vi "ClawGainScheduler.vi"(10 "On Bert?":bool=TRUE, 11 "Claw States":T2) -> (3 "ClawGainsOut":T1)   [LabVIEW 2014]
uses:
  Typedefs/ClawStates.ctl
panel:
  in  "Claw Gains for Ernie":T1={"Arm_kP"=13.5, "Arm_kI"=0.0, "Arm_kD"=0.0}
  in  "Claw Gains for Bert":T1={"Arm_kP"=10.0, "Arm_kI"=0.0, "Arm_kD"=0.0}
  in  "Claw Gains for Manual":T1
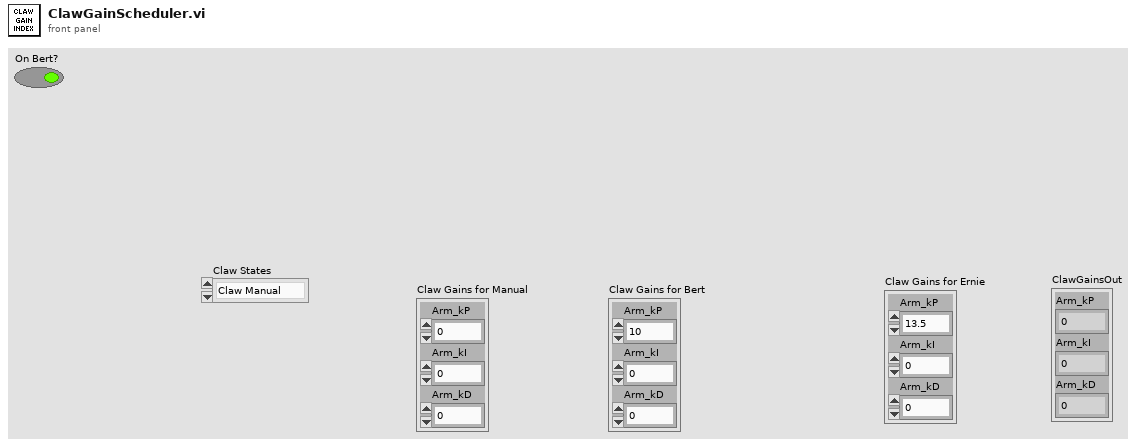
[diagram p1: front panel]
types:
  T1 = cluster{"Arm_kP":dbl, "Arm_kI":dbl, "Arm_kD":dbl}
  T2 = typedef "ClawStates.ctl" = enum16{"Claw Manual ", "Claw Open", "Claw Closed", "Claw Slight Open", "Flip Can"}
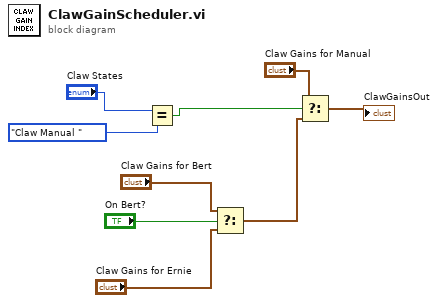
[diagram p0: block diagram]
diagram:
  n1 = Equal?(x="Claw States", y=ClawStates."Claw Manual " ("Claw States")) -> (x = y?=w6:bool)
  n2 = Select(t="Claw Gains for Bert", s="On Bert?", f="Claw Gains for Ernie") -> (s? t:f=w2:T1)
  n3 = Select(t="Claw Gains for Manual", s=w6, f=w2) -> (s? t:f=→"ClawGainsOut":T1)
